vi "Parameter XML Tx - Write.vi"(0 "String (in)":string, 7 "Parameter Array":T1[](array[typedef])) -> (4 "String (out)":string)   [LabVIEW 2017]
uses:
  Controls/Database_Array.ctl
  Controls/Encoding.ctl
  <userlib>/_OpenG.lib/array/array.llb/Remove Duplicates from 1D Array (I32)__ogtk.vi
  <userlib>/_OpenG.lib/array/array.llb/Filter 1D Array with Scalar (I32)__ogtk.vi
  <userlib>/_OpenG.lib/array/array.llb/Index 1D Array Elements (Variant)__ogtk.vi
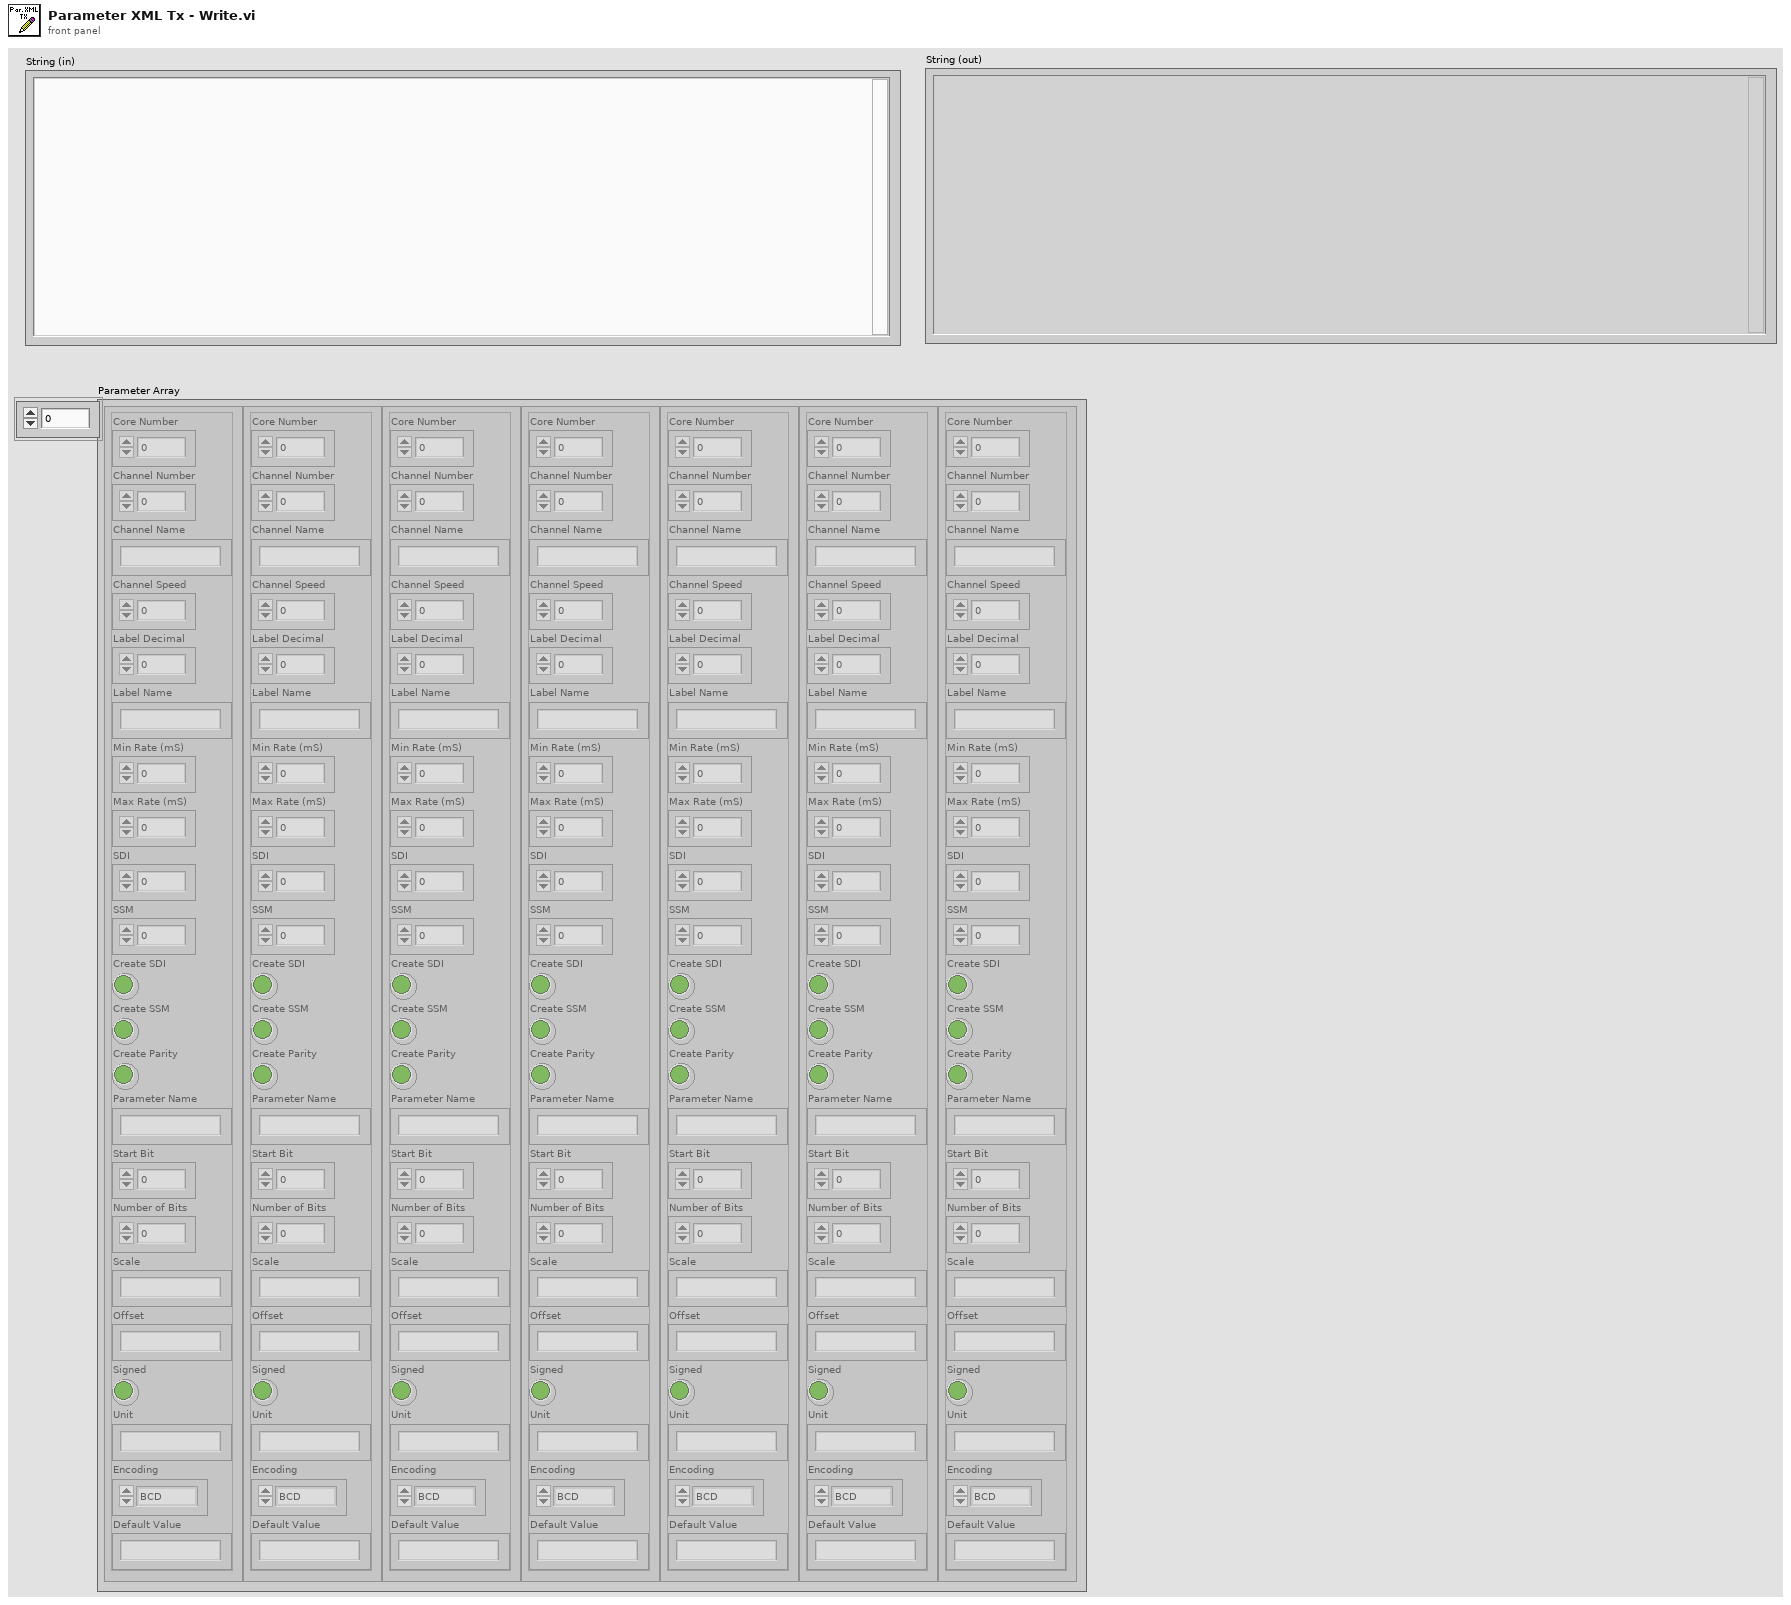
[diagram p1: front panel]
types:
  T1 = typedef "Database_Array.ctl" = cluster{"Core Number":i32, "Channel Number":i32, "Channel Name":string, "Channel Speed":i32, "Label Decimal":i32, "Label Name":string, "Min Rate (mS)":i32, "Max Rate (mS)":i32, "SDI":i32, "SSM":i32, "Create SDI":bool, "Create SSM":bool, "Create Parity":bool, "Parameter Name":string, "Start Bit":i32, "Number of Bits":i32, "Scale":string, "Offset":string, "Signed":bool, "Unit":string, "Encoding":T2, "Default Value":string}
  T2 = typedef "Encoding.ctl" = enum16{"BCD", "BNR", "Discrete"}
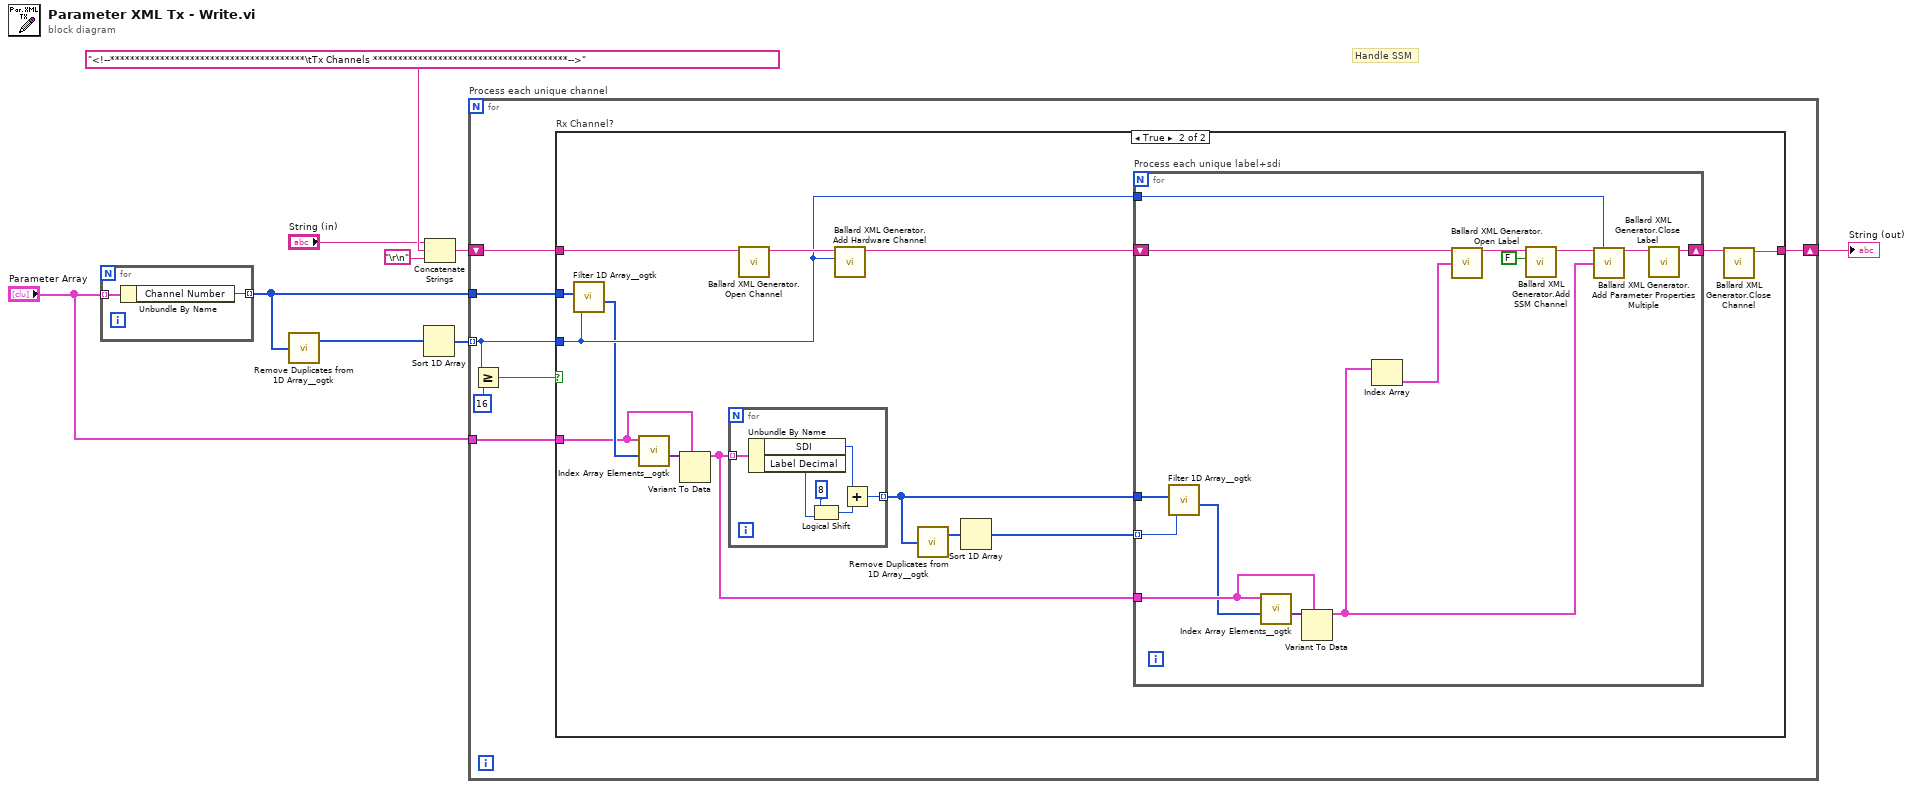
[diagram p0: block diagram]
diagram:
  # "Handle SSM"
  n1 = for {
    tunnel: [w11] -> w1 mode=indexing
    tunnel: "Parameter Array" -> [w10] mode=indexing
    n2 = Unbundle By Name(w10) -> ("Channel Number"=w11:i32)
  }
  n3 = call-poly <userlib>:"Remove Duplicates from 1D Array__ogtk.vi"("Input Array"=w1) -> ("Output Array"=w8:i32[])  [unwired: 1 out]
  n4 = Sort 1D Array(array=w8) -> (sorted array=w9:i32[])
  n5 = Concatenate Strings("String (in)", "<!--***************************************\tTx Channels ***************************************-->", "\r\n") -> (w5:string)
  n6 = for "Process each unique channel" {
    tunnel: w9 -> [w15] mode=indexing
    tunnel: w1 -> [w18]
    shift-right: [w16] -> w4
    shift-left: w5 -> [w17]
    tunnel: "Parameter Array" -> [w12]
    n7 = Greater Or Equal?(x=w15, y=16) -> (x >= y?=w14:bool)
    n8 = case "Rx Channel?" shown="True" w14 {
      tunnel: w18 -> [_ w33]
      tunnel: w17 -> [w19 w29]
      tunnel: [w19 w27] -> w16
      tunnel: w15 -> [_ w25]
      tunnel: w12 -> [_ w22]
      frame False {
      }
      frame True {
        n9 = call-poly <userlib>:"Filter 1D Array__ogtk.vi"("items to filter"=w25, "array"=w33) -> ("filtered item indices"=w23:i32[])  [unwired: 4 in, 1 out]
        n10 = call-poly <userlib>:"Index Array Elements__ogtk.vi"("indices"=w23, "array"=w22) -> ("elements"=w24:variant[])  [unwired: 9 in]
        n11 = Variant To Data(type=w22, Variant=w24) -> (data=w20:T1[])  [unwired: 1 in, 1 out]
        n12 = for {
          tunnel: w20 -> [w39] mode=indexing
          tunnel: [w34] -> w21 mode=indexing
          n13 = Unbundle By Name(w39) -> ("SDI"=w36:i32, "Label Decimal"=w35:i32)
          n14 = Logical Shift(y=i16 8, x=w35) -> (x << y=w38:i32)
          n15 = Add(x=w36, y=w38) -> (x+y=w34:i32)
        }
        n16 = call "Ballard XML Generator.Open Channel.vi"("string in"=w29) -> ("string out"=w30:string)  [unwired: 10 in]
        n17 = call "Ballard XML Generator.Add Hardware Channel.vi"("channel"=w25, "string in"=w30) -> ("string out"=w28:string)  [unwired: 9 in]
        n18 = call-poly <userlib>:"Remove Duplicates from 1D Array__ogtk.vi"("Input Array"=w21) -> ("Output Array"=w32:i32[])  [unwired: 1 out]
        n19 = Sort 1D Array(array=w32) -> (sorted array=w31:i32[])
        n20 = for "Process each unique label+sdi" {
          tunnel: w31 -> [w49] mode=indexing
          tunnel: w21 -> [w53]
          shift-right: [w48] -> w26
          shift-left: w28 -> [w50]
          tunnel: w25 -> [w42]
          tunnel: w20 -> [w44]
          n21 = call-poly <userlib>:"Filter 1D Array__ogtk.vi"("items to filter"=w49, "array"=w53) -> ("filtered item indices"=w43:i32[])  [unwired: 4 in, 1 out]
          n22 = call-poly <userlib>:"Index Array Elements__ogtk.vi"("indices"=w43, "array"=w44) -> ("elements"=w45:variant[])  [unwired: 9 in]
          n23 = Variant To Data(type=w44, Variant=w45) -> (data=w41:T1[])  [unwired: 1 in, 1 out]
          n24 = Index Array(array=w41) -> (element=w40:T1)  [unwired: 1 in]
          n25 = call "Ballard XML Generator.Open Label.vi"("string in"=w50, "input cluster"=w40) -> ("string out"=w52:string)  [unwired: 13 in]
          n26 = call "Ballard XML Generator.Add SSM Channel.vi"("create SSM chan?"=FALSE, "string in"=w52) -> ("string out"=w46:string)  [unwired: 9 in]
          n27 = call "Ballard XML Generator.Add Parameter Properties Multiple.vi"("string in"=w46, "Channel Number"=w42, "Parameter Array"=w41) -> ("string out"=w47:string)  [unwired: 12 in]
          n28 = call "Ballard XML Generator.Close Label.vi"("string in"=w47) -> ("string out"=w48:string)  [unwired: 10 in]
        }
        n29 = call "Ballard XML Generator.Close Channel.vi"("string in"=w26) -> ("string out"=w27:string)  [unwired: 10 in]
      }
    }
  }
  "String (out)" <- w4
